vi "Group_number_to_id.vi"(8 "error in (no error)":errorcluster, 11 "Group ID":i32) -> (0 "error out":errorcluster, 3 "Group name":string)   [LabVIEW 2011]
doc: "Displays a standard dialog box that prompts users to enter information, such as a user name and password.\n--------------------\n\nThis Express VI is configured as follows:\n\nMessage to Display to the User:Please Enter Experiment Settings Information For Database Storage.\nThe inputs are: \nNumber: Please Enter Group ID\nText Entry Box: Please Enter Tags:\nText Entry Box: Please Enter Experiment Description:"
uses:
  <vilib>/addons/database/Connection.llb/Conn Execute.vi
  <vilib>/addons/database/Recordset.llb/Rec Fetch Recordset Data (R).vi
  <vilib>/addons/database/Recordset.llb/Rec Destroy - Connection.vi
  <vilib>/addons/database/_DB Variant To Data/Database Variant To Data.xnode
  <vilib>/addons/database/NI_Database_API.lvlib
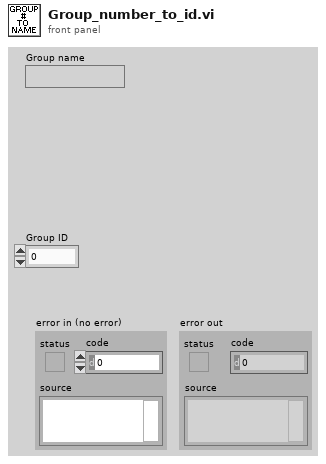
[diagram p1: front panel]
types:
  T1 = cluster{"Input Name":string, "Input Data Type":i32}
  T2 = typedef "NI_Database_API.lvlib/Conn ObjectReference.ctl" = refnum<k1>
  T3 = typedef "NI_Database_API.lvlib/Rec ObjectReference.ctl" = refnum<k1>
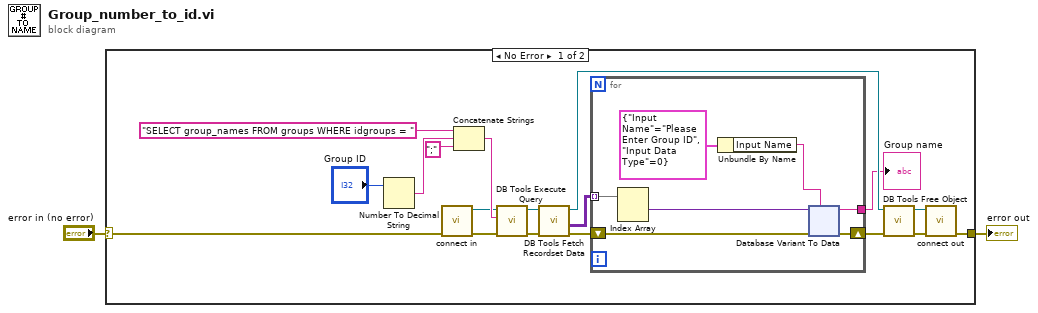
[diagram p0: block diagram]
diagram:
  n1 = case shown="No Error" "error in (no error)" {
    selector: "error in (no error)" -> [w20 w60]
    tunnel: [w11 w60] -> w1
    frame No Error {
      n2 = Number To Decimal String(number="Group ID") -> (decimal integer string=w9:string)  [unwired: 1 in]
      n3 = call "connect in.vi"("error in (no error)"=w20) -> ("error out"=w6:errorcluster, "Database Connection"=w5:T2)  [unwired: 6 in, 1 out]
      n4 = Concatenate Strings("SELECT group_names FROM groups WHERE idgroups = " ("SQL query"), w9, ";" ("string")) -> (w7:string)
      n5 = call-poly <vilib>:"DB Tools Execute Query.vi"("error in (no error)"=w6, "SQL query"=w7, "connection reference"=w5) -> ("error out"=w17:errorcluster, "recordset reference"=w16:T3)  [unwired: 5 in]
      n6 = call-poly <vilib>:"DB Tools Fetch Recordset Data.vi"("error in (no error)"=w17, "recordset reference"=w16) -> ("error out"=w19:errorcluster, "recordset data"=w18:variant[][], "recordset reference out"=w13:T3)  [unwired: 3 in]
      n7 = for {
        tunnel: w18 -> [w25] mode=indexing
        shift-right: [w21] -> w12
        shift-left: w19 -> [w24]
        tunnel: [w22] -> w4
        n8 = Index Array(array=w25) -> (element #1=w27:variant)  [unwired: 2 in, 1 out]
        n9 = Unbundle By Name(T1 {"Input Name"="Please Enter Group ID", "Input Data Type"=0}) -> ("Input Name"=w26:string)
        n10 = xnode "Database Variant To Data"("database variant"=w27, "error in"=w24, "type"=w26) -> ("data"=w22:string, "error out"=w21:errorcluster)
      }
      "Group name" <- w4
      n11 = call-poly <vilib>:"DB Tools Free Object.vi"("error in (no error)"=w12, "recordset reference"=w13) -> ("error out"=w14:errorcluster, "connection reference"=w15:T2)  [unwired: 8 in]
      n12 = call "connect out.vi"("error in (no error)"=w14, "connection reference"=w15) -> ("error out"=w11:errorcluster)  [unwired: 9 in]
    }
    frame Error {
    }
  }
  "error out" <- w1
